vi "_Serial_Mark10-Head_Moving.vi"(4 "Operation Mode":string(combo)="STOP", 5 "Serial Port":refnum<visa-resource-name>="COM5") -> (2 "VISA Resource name out":refnum<visa-resource-name>)   [LabVIEW 2015]
panel:
  # "MARK10 Control Head moving"
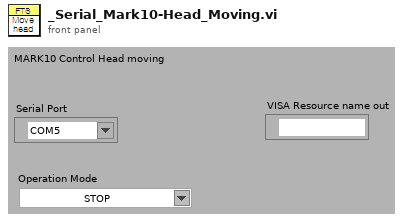
[diagram p1: front panel]
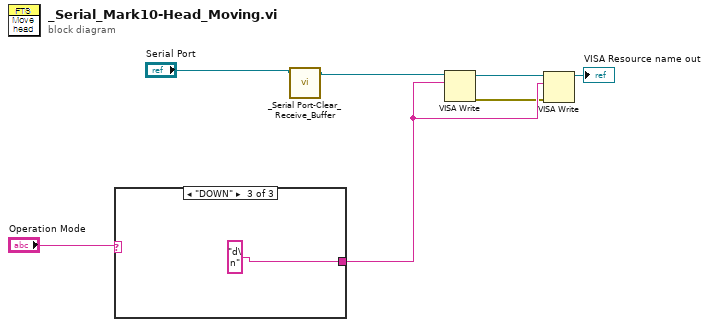
[diagram p0: block diagram]
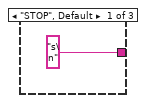
[diagram p2: hidden frame]
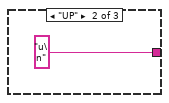
[diagram p3: hidden frame]
diagram:
  n1 = case shown="\"DOWN\"" "Operation Mode" {
    tunnel: ["s\n" "u\n" "d\n"] -> w5
    frame "STOP", Default {
    }
    frame "UP" {
    }
    frame "DOWN" {
    }
  }
  n2 = call "_Serial Port-Clear_Receive_Buffer.vi"("Serial Port"="Serial Port") -> ("Serial Port out"=w1:refnum<visa-resource-name>)  [unwired: 3 in, 1 out]
  n3 = VISA Write(VISA resource name=w1, write buffer=w5) -> (VISA resource name out=w6:refnum<visa-resource-name>, error out=w4:errorcluster)  [unwired: 1 in, 1 out]
  n4 = VISA Write(VISA resource name=w6, write buffer=w5, error in (no error)=w4) -> (VISA resource name out=→"VISA Resource name out":refnum<visa-resource-name>)  [unwired: 2 out]
